vi "ClassInit.vi"(8 "error in (no error)":errorcluster, 10 "data":T1) -> (0 "error out":errorcluster, 3 "Execute":refnum<class "Execute.lvclass">)   [LabVIEW 2018, in "QMH_Class.lvlib" / "TestManager.lvlib" / "Execute.lvclass"]
uses:
  Execute.lvclass
  Execute.lvclass/Execute.ctl
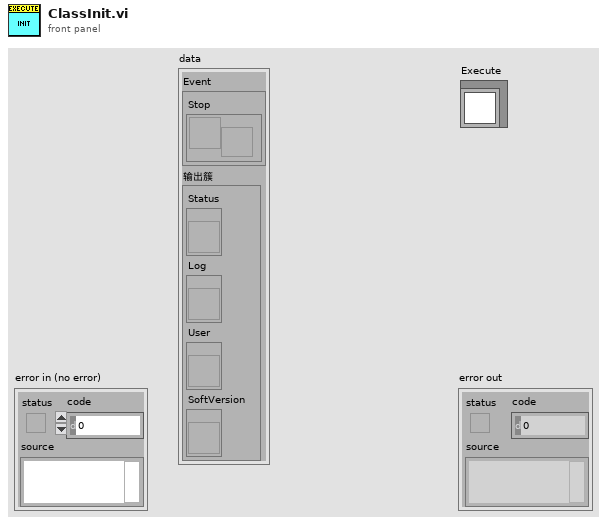
[diagram p1: front panel]
types:
  T1 = cluster{"Event":cluster{"Stop":refnum<user-event>}, "输出簇":cluster{"Status":refnum<vi>, "Log":refnum<vi>, "User":refnum<vi>, "SoftVersion":refnum<vi>}}
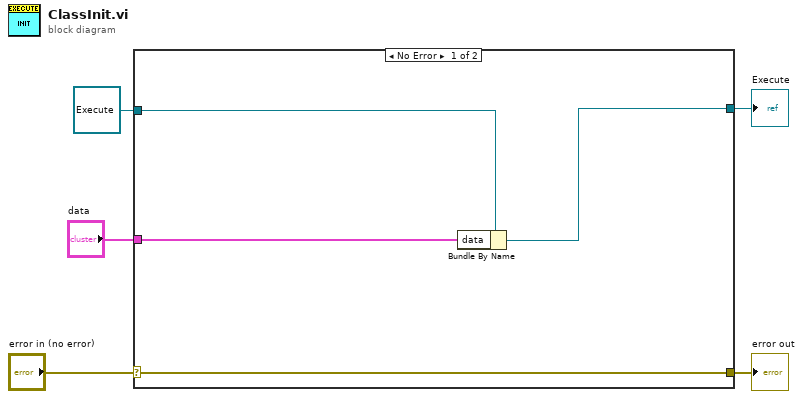
[diagram p0: block diagram]
diagram:
  n1 = case shown="No Error" "error in (no error)" {
    selector: "error in (no error)" -> [w8 w11]
    tunnel: [w8 w11] -> w4
    tunnel: [w9 w10] -> w3
    tunnel: "data" -> [w7 _]
    tunnel: refnum<class "Execute.lvclass"> refnum ("QMH_Class.lvlib:TestManager.lvlib:Execute.lvclass") -> [w6 w10]
    frame No Error {
      n2 = Bundle By Name(cluster=w6, "data"=w7) -> (w9:refnum<class "Execute.lvclass">)
    }
    frame Error {
    }
  }
  "error out" <- w4
  "Execute" <- w3
